vi "Test_Multiple_SubPanel_Self HSMO_External_Control.vi"() -> ()   [LabVIEW 2021]
uses:
  C:/Program Files (x86)/Hyper State Machine Framework/SSW_Hyper_State_Machine.lvlibp/State_Machine_Class/Main_State_Machine/Hyper_State_Machine.lvclass
  C:/Program Files (x86)/Hyper State Machine Framework/SSW_Hyper_State_Machine.lvlibp/State_Machine_Class/State_Machine_Module.llb/State Machine.ctl
  C:/Program Files (x86)/Hyper State Machine Framework/SSW_Hyper_State_Machine.lvlibp
panel:
  in  "Panel Index":i32
  in  "Change Mode":bool=TRUE
  out "Total_State":i32 caption="Total Independent State Object"
  in  "Show Stop Button":bool
  in  "UnLoad_Panel":bool
  in  "Load_Panel":bool
  in  "Time Target (s)":dbl=30.0 format="%#_13g"
  in  "System_Delay(s)":dbl=0.01 format="%.0p"
  in  "State_Interval_Time(s)":dbl format="%.0p"
  in  "State#":i32=100
  in  "Stop":bool=TRUE
  out "State[]":refnum<class "Hyper_State_Machine.lvclass">[][](array[class])
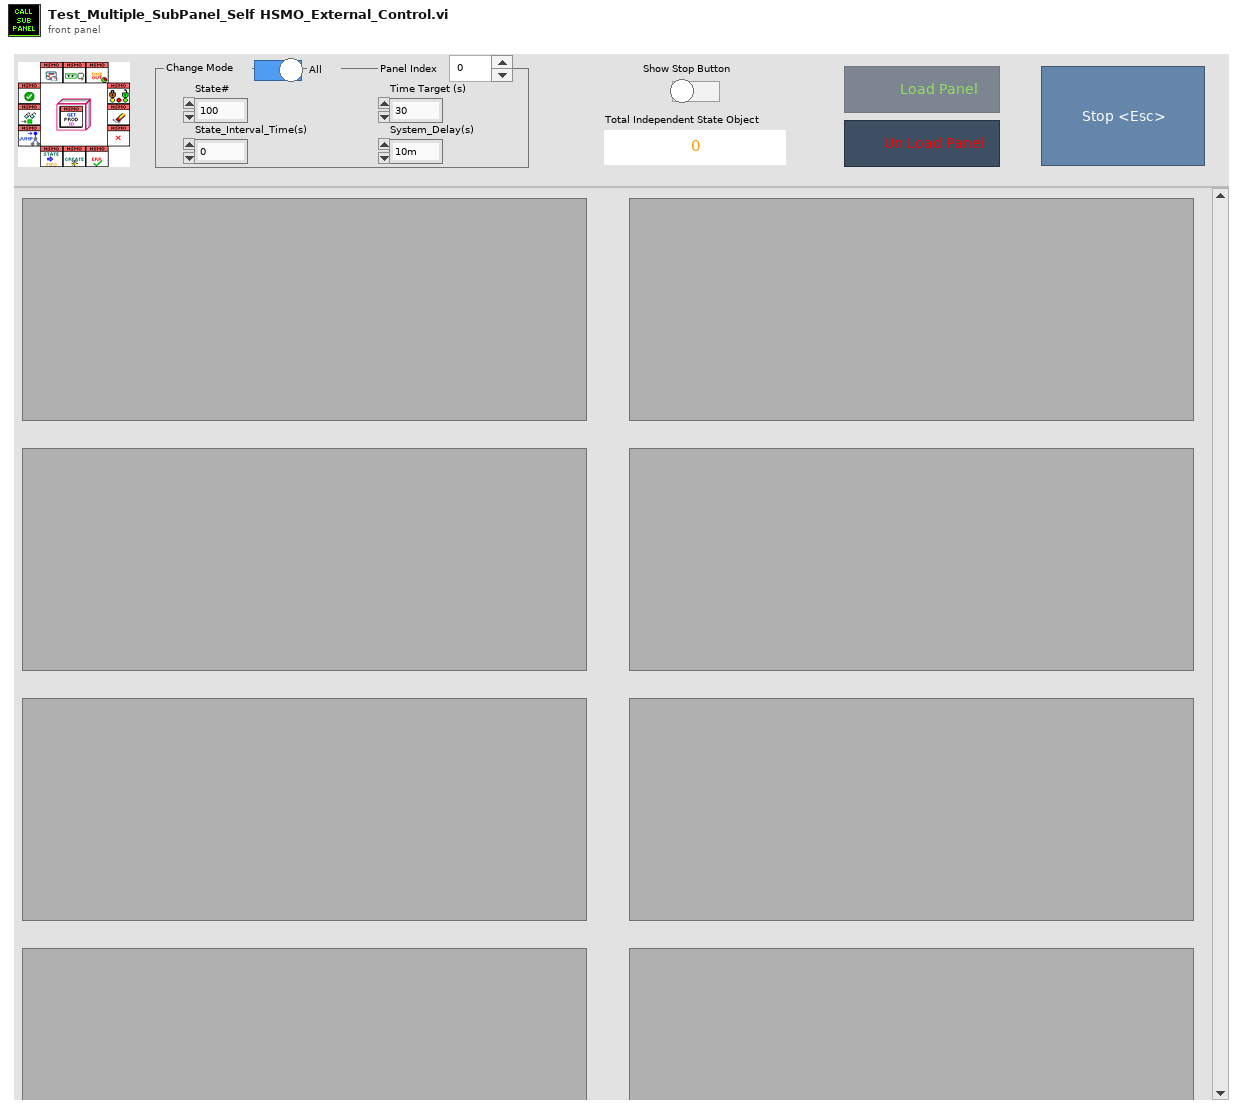
[diagram p1: front panel]
types:
  T1 = enum8{"Enabled", "Disabled", "Disabled and Grayed Out"}
  T2 = typedef "SSW_Hyper_State_Machine.lvlibp/State Machine.ctl" = cluster{"Command":string, "Data":variant}
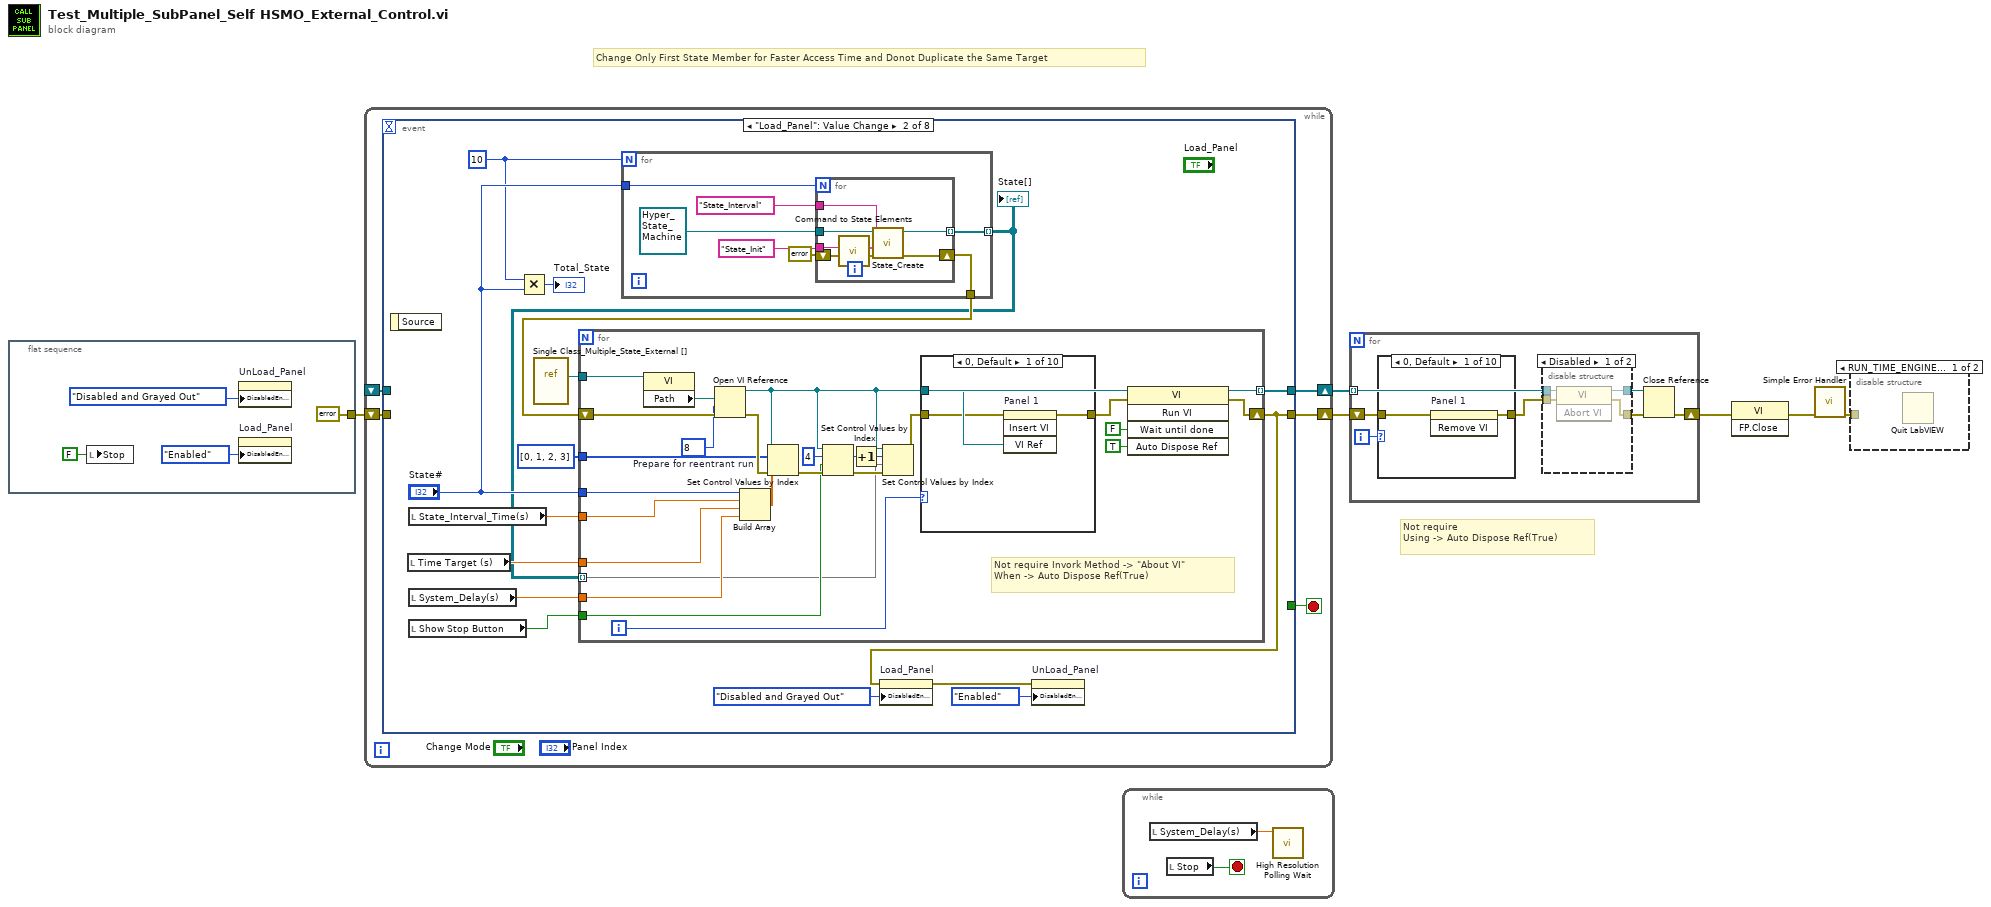
[diagram p0: block diagram]
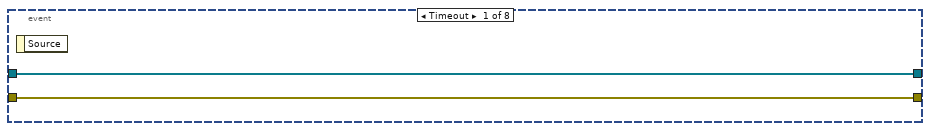
[diagram p3: hidden frame]
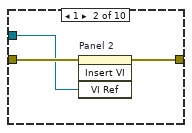
[diagram p4: hidden frame]
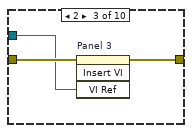
[diagram p5: hidden frame]
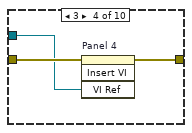
[diagram p6: hidden frame]
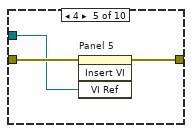
[diagram p7: hidden frame]
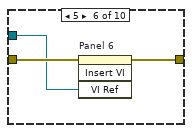
[diagram p8: hidden frame]
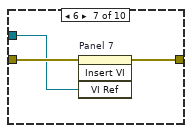
[diagram p9: hidden frame]
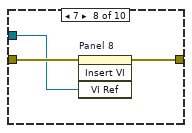
[diagram p10: hidden frame]
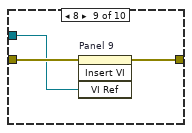
[diagram p11: hidden frame]
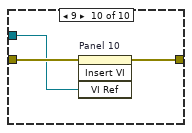
[diagram p12: hidden frame]
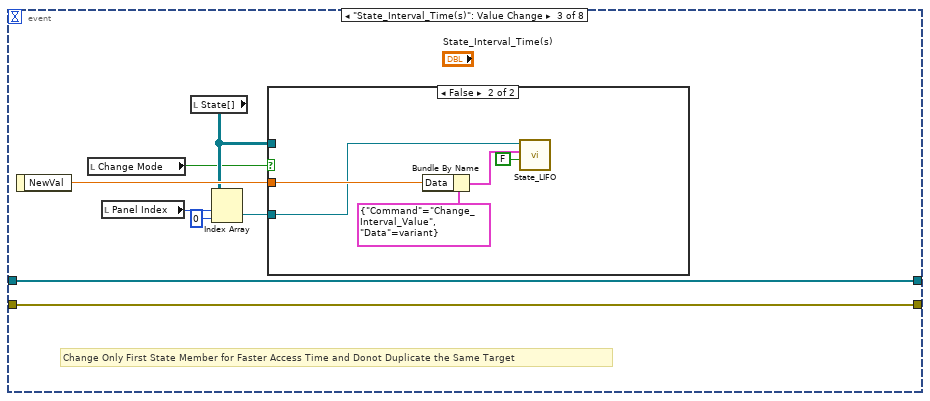
[diagram p13: hidden frame]
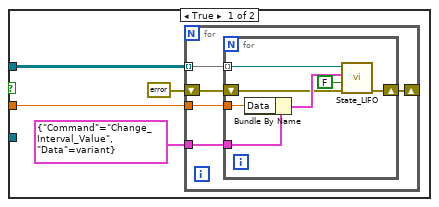
[diagram p14: hidden frame]
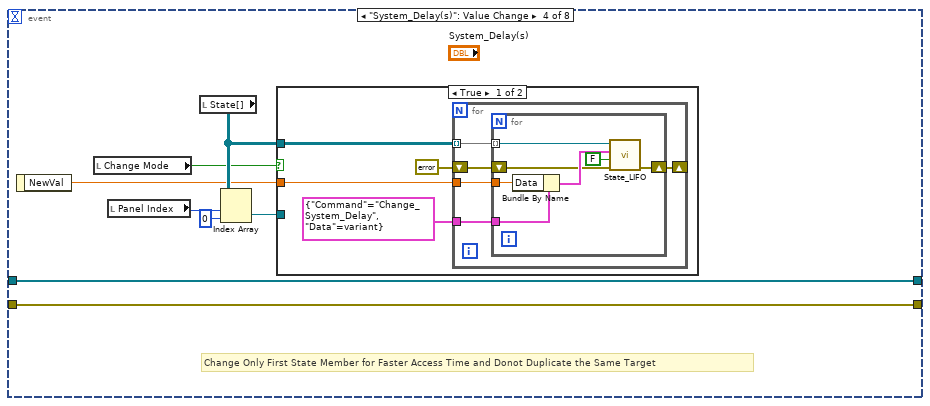
[diagram p15: hidden frame]
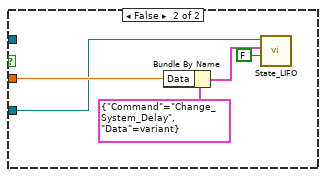
[diagram p16: hidden frame]
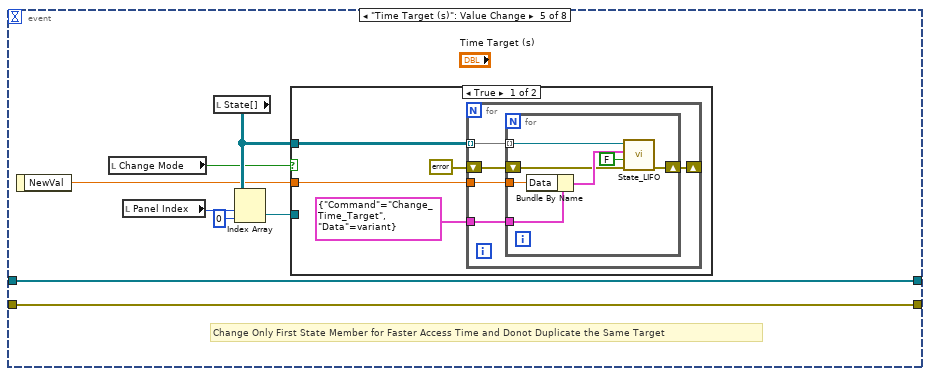
[diagram p17: hidden frame]
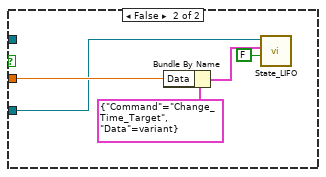
[diagram p18: hidden frame]
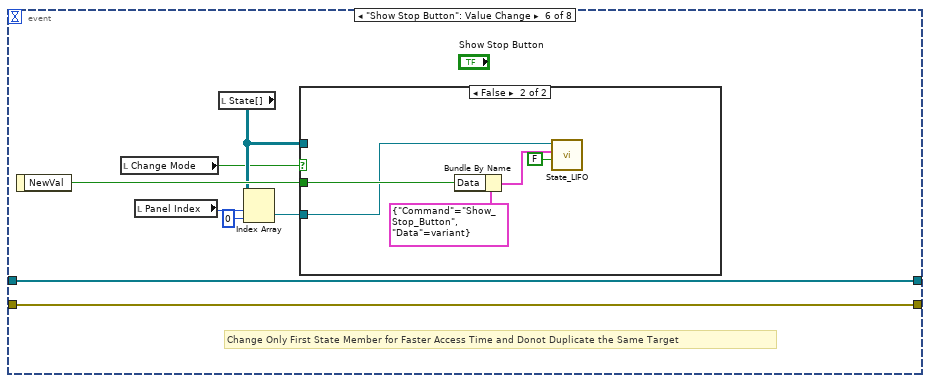
[diagram p19: hidden frame]
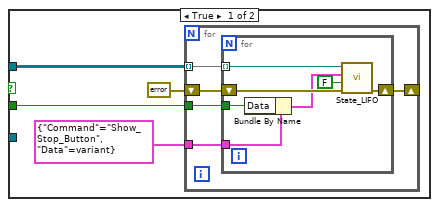
[diagram p20: hidden frame]
diagram:
  # "Change Only First State Member for Faster Access Time and Donot Duplicate the Same Target"
  # "Not require\nUsing -> Auto Dispose Ref(True)"
  n1 = flat-sequence {
    tunnel: [errorcluster {"status"=FALSE, "code"=0, "source"=""} ("error out")] -> w4
    frame #0 {
      n2 = local write "Stop"(FALSE ("Stop")) -> ()
      n3 = property on="UnLoad_Panel" class="Bool"("DisabledEnum"=T1."Disabled and Grayed Out" ("Disabled")) -> ()  [unwired: 2 in, 2 out]
      n4 = property on="Load_Panel" class="Bool"("DisabledEnum"=T1."Enabled" ("Disabled")) -> ()  [unwired: 2 in, 2 out]
    }
  }
  n5 = while {
    shift-right: [w14] -> w6
    shift-left: _ -> [w13]
    shift-right: [w12] -> w5
    shift-left: w4 -> [w11]
    stop <- w15 stop-if-true
    n6 = event shown="[1] \"Load_Panel\": Value Change" {
      selector: _ -> [_ _ _ _ _ _ _ _]
      dyn-events: _ -> [_ _ _ _ _ _ _ _]
      timeout: _ -> [_ _ _ _ _ _ _ _]
      tunnel: [_ _ _ _ _ _ _ w259] -> w15
      tunnel: [w17 w32 w109 w139 w168 w197 _ w260] -> w14
      tunnel: w13 -> [w17 _ w109 w139 w168 w197 w224 w260]
      tunnel: [w16 w28 w108 w138 w167 w196 _ w258] -> w12
      tunnel: w11 -> [w16 _ w108 w138 w167 w196 w220 w258]
      event Timeout {
        n7 = event-data() -> ()  [unwired: 1 in, 1 out]
      }
      event "Load_Panel": Value Change {
        w23 = 10
        n8 = event-data() -> ()  [unwired: 1 in, 1 out]
        n9 = local read "Time Target (s)"() -> (w20:dbl)
        n10 = local read "State_Interval_Time(s)"() -> (w26:dbl)
        n11 = local read "System_Delay(s)"() -> (w22:dbl)
        n12 = local read "Show Stop Button"() -> (w21:bool)
        n13 = Multiply(x=w23, y="State#") -> (x*y=→"Total_State":i32)
        n14 = vi-ref "Single Class_Multiple_State_External [].vi"() -> (w18:refnum<vi>)
        n15 = for {
          N: w23 -> [_]
          tunnel: [w36] -> w25
          tunnel: "State#" -> [w35]
          tunnel: [w34] -> w19 mode=indexing
          n16 = for {
            N: w35 -> [_]
            tunnel: refnum<class "Hyper_State_Machine.lvclass"> refnum ("SSW_Hyper_State_Machine.lvlibp:Hyper_State_Machine.lvclass") -> [w47]
            tunnel: "State_Init" ("Command") -> [w45]
            tunnel: "State_Interval" ("Core_Interval_Name(State_Interval)") -> [w44]
            shift-right: [w43] -> w36
            shift-left: errorcluster {"status"=FALSE, "code"=0, "source"=""} ("error out") -> [w42]
            tunnel: [w41] -> w34 mode=indexing
            n17 = call "Command to State Elements.vi"("Command"=w45) -> ("Command to State Elements"=w46:T2)  [unwired: 10 in]
            n18 = call-dynamic "State_Create.vi"("error in (no error)"=w42, "Init_State(Option)"=w46, "State_Interval_Name"=w44, "State_Machine_Class in"=w47) -> ("error out"=w43:errorcluster, "State_Machine_Class out"=w41:refnum<class "Hyper_State_Machine.lvclass">)  [unwired: 5 in, 1 out]
          }
        }
        "State[]" <- w19
        n19 = for {
          shift-right: [w65] -> w28
          shift-left: w25 -> [w71]
          tunnel: [w67] -> w32 mode=indexing
          tunnel: w26 -> [w62]
          tunnel: "State#" -> [w61]
          tunnel: w22 -> [w60]
          tunnel: w20 -> [w59]
          tunnel: i32[] [0, 1, 2, 3] ("control indexes") -> [w58]
          tunnel: w21 -> [w57]
          tunnel: w19 -> [w50] mode=indexing
          tunnel: w18 -> [w48]
          i -> [w51]
          w54 = 4
          w49 = 8  # Prepare for reentrant run
          # "Not require Invork Method -> \"About VI\"\nWhen -> Auto Dispose Ref(True)"
          n20 = property class="VI"(reference=w48) -> ("Path"=w72:path)  [unwired: 1 in, 2 out]
          n21 = Open VI Reference(vi path=w72, options=w49, error in (no error)=w71) -> (vi reference=w52:refnum<vi>, error out=w70:errorcluster)  [unwired: 3 in]
          n22 = Build Array(w61, w62, w59, w60) -> (w64:dbl[])
          n23 = Set Control Values by Index(0:w52, 1:w58, 2:w64, 3:w70) -> (11:w63:errorcluster)
          n24 = Set Control Values by Index(0:w52, 1:w54, 2:w57, 3:w63) -> (11:w56:errorcluster)
          n25 = Increment(x=w54) -> (x+1=w53:i32)
          n26 = Set Control Values by Index(0:w52, 1:w53, 2:w50, 3:w56) -> (11:w55:errorcluster)
          n27 = case shown="0, Default" w51 {
            tunnel: w55 -> [w73 w78 w81 w84 w87 w90 w93 w96 w99 w102]
            tunnel: w52 -> [w74 w77 w79 w82 w85 w88 w91 w94 w97 w100]
            tunnel: [w75 w76 w80 w83 w86 w89 w92 w95 w98 w101] -> w66
            frame 0, Default {
              n28 = invoke on="Panel 1" class="SubPnl" method="Insert VI"(error in=w73, "VI Ref"=w74) -> (error out=w75:errorcluster)  [unwired: 2 in, 3 out]
            }
            frame 1 {
              n29 = invoke on="Panel 2" class="SubPnl" method="Insert VI"(error in=w78, "VI Ref"=w77) -> (error out=w76:errorcluster)  [unwired: 2 in, 3 out]
            }
            frame 2 {
              n30 = invoke on="Panel 3" class="SubPnl" method="Insert VI"(error in=w81, "VI Ref"=w79) -> (error out=w80:errorcluster)  [unwired: 2 in, 3 out]
            }
            frame 3 {
              n31 = invoke on="Panel 4" class="SubPnl" method="Insert VI"(error in=w84, "VI Ref"=w82) -> (error out=w83:errorcluster)  [unwired: 2 in, 3 out]
            }
            frame 4 {
              n32 = invoke on="Panel 5" class="SubPnl" method="Insert VI"(error in=w87, "VI Ref"=w85) -> (error out=w86:errorcluster)  [unwired: 2 in, 3 out]
            }
            frame 5 {
              n33 = invoke on="Panel 6" class="SubPnl" method="Insert VI"(error in=w90, "VI Ref"=w88) -> (error out=w89:errorcluster)  [unwired: 2 in, 3 out]
            }
            frame 6 {
              n34 = invoke on="Panel 7" class="SubPnl" method="Insert VI"(error in=w93, "VI Ref"=w91) -> (error out=w92:errorcluster)  [unwired: 2 in, 3 out]
            }
            frame 7 {
              n35 = invoke on="Panel 8" class="SubPnl" method="Insert VI"(error in=w96, "VI Ref"=w94) -> (error out=w95:errorcluster)  [unwired: 2 in, 3 out]
            }
            frame 8 {
              n36 = invoke on="Panel 9" class="SubPnl" method="Insert VI"(error in=w99, "VI Ref"=w97) -> (error out=w98:errorcluster)  [unwired: 2 in, 3 out]
            }
            frame 9 {
              n37 = invoke on="Panel 10" class="SubPnl" method="Insert VI"(error in=w102, "VI Ref"=w100) -> (error out=w101:errorcluster)  [unwired: 2 in, 3 out]
            }
          }
          n38 = invoke class="VI" method="Run VI"(reference=w52, error in=w66, "Wait until done"=FALSE ("Wait Until Done"), "Auto Dispose Ref"=TRUE ("Auto Dispose Reference")) -> (reference out=w67:refnum<vi>, error out=w65:errorcluster)  [unwired: 1 in, 3 out]
        }
        n39 = property on="Load_Panel" class="Bool"(error in=w28, "DisabledEnum"=T1."Disabled and Grayed Out" ("Disabled")) -> (error out=w29:errorcluster)  [unwired: 1 in, 1 out]
        n40 = property on="UnLoad_Panel" class="Bool"(error in=w29, "DisabledEnum"=T1."Enabled" ("Disabled")) -> ()  [unwired: 1 in, 2 out]
      }
      event "State_Interval_Time(s)": Value Change {
        # "Change Only First State Member for Faster Access Time and Donot Duplicate the Same Target"
        n41 = event-data() -> ("NewVal"=w110:dbl)  [unwired: 1 in]
        n42 = local read "Change Mode"() -> (w104:bool)
        n43 = local read "Panel Index"() -> (w103:i32)
        n44 = local read "State[]"() -> (w107:refnum<class "Hyper_State_Machine.lvclass">[][])
        n45 = Index Array(array=w107, index (row)=w103, index (col)=0 ("disabled index (col)")) -> (element=w106:refnum<class "Hyper_State_Machine.lvclass">)
        n46 = case shown="False" w104 {
          tunnel: w110 -> [w114 w131]
          tunnel: w107 -> [w111 _]
          tunnel: w106 -> [_ w130]
          frame True {
            n47 = for {
              tunnel: w111 -> [w119] mode=indexing
              shift-right: [w116] -> _
              shift-left: errorcluster {"status"=FALSE, "code"=0, "source"=""} ("error out") -> [w117]
              tunnel: w114 -> [w118]
              tunnel: T2 {"Command"="Change_Interval_Value", "Data"=variant} ("State Machine") -> [w115]
              n48 = for {
                tunnel: w119 -> [w122] mode=indexing
                tunnel: w118 -> [w125]
                shift-right: [w124] -> w116
                shift-left: w117 -> [w121]
                tunnel: w115 -> [w123]
                n49 = Bundle By Name(cluster=w123, "Data"=w125) -> (w126:T2)
                n50 = call-dynamic "State_LIFO.vi"("error in (no error)"=w121, "State_Interval(Enable)"=FALSE, "State Machine"=w126, "State_Machine_Class in"=w122) -> ("error out"=w124:errorcluster)  [unwired: 6 in, 1 out]
              }
            }
          }
          frame False {
            n51 = Bundle By Name(cluster=T2 {"Command"="Change_Interval_Value", "Data"=variant} ("State Machine"), "Data"=w131) -> (w128:T2)
            n52 = call-dynamic "State_LIFO.vi"("State_Interval(Enable)"=FALSE, "State Machine"=w128, "State_Machine_Class in"=w130) -> ()  [unwired: 7 in, 2 out]
          }
        }
      }
      event "System_Delay(s)": Value Change {
        # "Change Only First State Member for Faster Access Time and Donot Duplicate the Same Target"
        n53 = event-data() -> ("NewVal"=w135:dbl)  [unwired: 1 in]
        n54 = local read "Change Mode"() -> (w133:bool)
        n55 = local read "Panel Index"() -> (w132:i32)
        n56 = local read "State[]"() -> (w137:refnum<class "Hyper_State_Machine.lvclass">[][])
        n57 = Index Array(array=w137, index (row)=w132, index (col)=0 ("disabled index (col)")) -> (element=w136:refnum<class "Hyper_State_Machine.lvclass">)
        n58 = case shown="True" w133 {
          tunnel: w135 -> [w143 w160]
          tunnel: w137 -> [w140 _]
          tunnel: w136 -> [_ w159]
          frame True {
            n59 = for {
              tunnel: w140 -> [w148] mode=indexing
              shift-right: [w145] -> _
              shift-left: errorcluster {"status"=FALSE, "code"=0, "source"=""} ("error out") -> [w146]
              tunnel: w143 -> [w147]
              tunnel: T2 {"Command"="Change_System_Delay", "Data"=variant} ("State Machine") -> [w144]
              n60 = for {
                tunnel: w148 -> [w151] mode=indexing
                tunnel: w147 -> [w154]
                shift-right: [w153] -> w145
                shift-left: w146 -> [w150]
                tunnel: w144 -> [w152]
                n61 = Bundle By Name(cluster=w152, "Data"=w154) -> (w155:T2)
                n62 = call-dynamic "State_LIFO.vi"("error in (no error)"=w150, "State_Interval(Enable)"=FALSE, "State Machine"=w155, "State_Machine_Class in"=w151) -> ("error out"=w153:errorcluster)  [unwired: 6 in, 1 out]
              }
            }
          }
          frame False {
            n63 = Bundle By Name(cluster=T2 {"Command"="Change_System_Delay", "Data"=variant} ("State Machine"), "Data"=w160) -> (w157:T2)
            n64 = call-dynamic "State_LIFO.vi"("State_Interval(Enable)"=FALSE, "State Machine"=w157, "State_Machine_Class in"=w159) -> ()  [unwired: 7 in, 2 out]
          }
        }
      }
      event "Time Target (s)": Value Change {
        # "Change Only First State Member for Faster Access Time and Donot Duplicate the Same Target"
        n65 = event-data() -> ("NewVal"=w164:dbl)  [unwired: 1 in]
        n66 = local read "Change Mode"() -> (w162:bool)
        n67 = local read "Panel Index"() -> (w161:i32)
        n68 = local read "State[]"() -> (w166:refnum<class "Hyper_State_Machine.lvclass">[][])
        n69 = Index Array(array=w166, index (row)=w161, index (col)=0 ("disabled index (col)")) -> (element=w165:refnum<class "Hyper_State_Machine.lvclass">)
        n70 = case shown="True" w162 {
          tunnel: w164 -> [w172 w189]
          tunnel: w166 -> [w169 _]
          tunnel: w165 -> [_ w188]
          frame True {
            n71 = for {
              tunnel: w169 -> [w177] mode=indexing
              shift-right: [w174] -> _
              shift-left: errorcluster {"status"=FALSE, "code"=0, "source"=""} ("error out") -> [w175]
              tunnel: w172 -> [w176]
              tunnel: T2 {"Command"="Change_Time_Target", "Data"=variant} ("State Machine") -> [w173]
              n72 = for {
                tunnel: w177 -> [w180] mode=indexing
                tunnel: w176 -> [w183]
                shift-right: [w182] -> w174
                shift-left: w175 -> [w179]
                tunnel: w173 -> [w181]
                n73 = Bundle By Name(cluster=w181, "Data"=w183) -> (w184:T2)
                n74 = call-dynamic "State_LIFO.vi"("error in (no error)"=w179, "State_Interval(Enable)"=FALSE, "State Machine"=w184, "State_Machine_Class in"=w180) -> ("error out"=w182:errorcluster)  [unwired: 6 in, 1 out]
              }
            }
          }
          frame False {
            n75 = Bundle By Name(cluster=T2 {"Command"="Change_Time_Target", "Data"=variant} ("State Machine"), "Data"=w189) -> (w186:T2)
            n76 = call-dynamic "State_LIFO.vi"("State_Interval(Enable)"=FALSE, "State Machine"=w186, "State_Machine_Class in"=w188) -> ()  [unwired: 7 in, 2 out]
          }
        }
      }
      event "Show Stop Button": Value Change {
        # "Change Only First State Member for Faster Access Time and Donot Duplicate the Same Target"
        n77 = event-data() -> ("NewVal"=w194:bool)  [unwired: 1 in]
        n78 = local read "Change Mode"() -> (w191:bool)
        n79 = local read "Panel Index"() -> (w190:i32)
        n80 = local read "State[]"() -> (w192:refnum<class "Hyper_State_Machine.lvclass">[][])
        n81 = Index Array(array=w192, index (row)=w190, index (col)=0 ("disabled index (col)")) -> (element=w195:refnum<class "Hyper_State_Machine.lvclass">)
        n82 = case shown="False" w191 {
          tunnel: w194 -> [w201 w218]
          tunnel: w195 -> [_ w217]
          tunnel: w192 -> [w198 _]
          frame True {
            n83 = for {
              tunnel: w198 -> [w206] mode=indexing
              shift-right: [w203] -> _
              shift-left: errorcluster {"status"=FALSE, "code"=0, "source"=""} ("error out") -> [w204]
              tunnel: w201 -> [w205]
              tunnel: T2 {"Command"="Show_Stop_Button", "Data"=variant} ("State Machine") -> [w202]
              n84 = for {
                tunnel: w206 -> [w213] mode=indexing
                tunnel: w205 -> [w212]
                tunnel: w202 -> [w209]
                shift-right: [w210] -> w203
                shift-left: w204 -> [w211]
                n85 = Bundle By Name(cluster=w209, "Data"=w212) -> (w208:T2)
                n86 = call-dynamic "State_LIFO.vi"("error in (no error)"=w211, "State_Interval(Enable)"=FALSE, "State Machine"=w208, "State_Machine_Class in"=w213) -> ("error out"=w210:errorcluster)  [unwired: 6 in, 1 out]
              }
            }
          }
          frame False {
            n87 = Bundle By Name(cluster=T2 {"Command"="Show_Stop_Button", "Data"=variant} ("State Machine"), "Data"=w218) -> (w215:T2)
            n88 = call-dynamic "State_LIFO.vi"("State_Interval(Enable)"=FALSE, "State Machine"=w215, "State_Machine_Class in"=w217) -> ()  [unwired: 7 in, 2 out]
          }
        }
      }
      event "UnLoad_Panel": Value Change {
        # "Do not using Shift Register to ignore some case Error"
        # "Not require\nUsing -> Auto Dispose Ref(True)"
        n89 = event-data() -> ()  [unwired: 1 in, 1 out]
        n90 = for {
          tunnel: w224 -> [w229] mode=indexing
          tunnel: w220 -> [w226]
          tunnel: [w225] -> w219
          i -> [w228]
          n91 = case shown="0, Default" w228 {
            tunnel: w226 -> [w238 w241 w243 w245 w247 w249 w251 w253 w255 w257]
            tunnel: w229 -> [_ _ _ _ _ _ _ _ _ _]
            tunnel: [w239 w240 w242 w244 w246 w248 w250 w252 w254 w256] -> w227
            frame 0, Default {
              n92 = invoke on="Panel 1" class="SubPnl" method="Remove VI"(error in=w238) -> (error out=w239:errorcluster)  [unwired: 2 in, 2 out]
            }
            frame 1 {
              n93 = invoke on="Panel 2" class="SubPnl" method="Remove VI"(error in=w241) -> (error out=w240:errorcluster)  [unwired: 2 in, 2 out]
            }
            frame 2 {
              n94 = invoke on="Panel 3" class="SubPnl" method="Remove VI"(error in=w243) -> (error out=w242:errorcluster)  [unwired: 2 in, 2 out]
            }
            frame 3 {
              n95 = invoke on="Panel 4" class="SubPnl" method="Remove VI"(error in=w245) -> (error out=w244:errorcluster)  [unwired: 2 in, 2 out]
            }
            frame 4 {
              n96 = invoke on="Panel 5" class="SubPnl" method="Remove VI"(error in=w247) -> (error out=w246:errorcluster)  [unwired: 2 in, 2 out]
            }
            frame 5 {
              n97 = invoke on="Panel 6" class="SubPnl" method="Remove VI"(error in=w249) -> (error out=w248:errorcluster)  [unwired: 2 in, 2 out]
            }
            frame 6 {
              n98 = invoke on="Panel 7" class="SubPnl" method="Remove VI"(error in=w251) -> (error out=w250:errorcluster)  [unwired: 2 in, 2 out]
            }
            frame 7 {
              n99 = invoke on="Panel 8" class="SubPnl" method="Remove VI"(error in=w253) -> (error out=w252:errorcluster)  [unwired: 2 in, 2 out]
            }
            frame 8 {
              n100 = invoke on="Panel 9" class="SubPnl" method="Remove VI"(error in=w255) -> (error out=w254:errorcluster)  [unwired: 2 in, 2 out]
            }
            frame 9 {
              n101 = invoke on="Panel 10" class="SubPnl" method="Remove VI"(error in=w257) -> (error out=w256:errorcluster)  [unwired: 2 in, 2 out]
            }
          }
          n102 = disable-structure shown="Enabled" {
            disable-tunnel: [w235 w237] -> w231
            disable-tunnel: [w234 w236] -> w230
            disable-tunnel: w229 -> [w233 w237]
            disable-tunnel: w227 -> [w232 w236]
            frame Disabled {
              n103 = invoke class="VI" method="Abort VI"(reference=w233, error in=w232) -> (reference out=w235:refnum<vi>, error out=w234:errorcluster)  [unwired: 1 in, 1 out]
            }
            frame Enabled {
            }
          }
          n104 = Close Reference(reference=w231, error in (no error)=w230) -> (error out=w225:errorcluster)
        }
        n105 = property on="UnLoad_Panel" class="Bool"(error in=w219, "DisabledEnum"=T1."Disabled and Grayed Out" ("Disabled")) -> (error out=w221:errorcluster)  [unwired: 1 in, 1 out]
        n106 = property on="Load_Panel" class="Bool"(error in=w221, "DisabledEnum"=T1."Enabled" ("Disabled")) -> ()  [unwired: 1 in, 2 out]
      }
      event "Stop": Value Change {
        n107 = event-data() -> ()  [unwired: 1 in, 1 out]
        n108 = Two Button Dialog(message="Exit Confirm !") -> (T button?=w259:bool)  [unwired: 2 in]
        n109 = local write "Stop"(w259) -> ()
      }
    }
  }
  n110 = while {
    stop <- w262 stop-if-true
    n111 = local read "System_Delay(s)"() -> (w263:dbl)
    n112 = local read "Stop"() -> (w262:bool)
    n113 = call <vilib>:"High Resolution Polling Wait.vi"("seconds to wait"=w263) -> ()  [unwired: 10 in, 1 out]
  }
  n114 = for {
    tunnel: w6 -> [w270] mode=indexing
    shift-right: [w267] -> w2
    shift-left: w5 -> [w266]
    i -> [w265]
    n115 = case shown="0, Default" w265 {
      tunnel: w266 -> [w277 w280 w282 w284 w286 w288 w290 w292 w294 w296]
      tunnel: [w278 w279 w281 w283 w285 w287 w289 w291 w293 w295] -> w264
      frame 0, Default {
        n116 = invoke on="Panel 1" class="SubPnl" method="Remove VI"(error in=w277) -> (error out=w278:errorcluster)  [unwired: 2 in, 2 out]
      }
      frame 1 {
        n117 = invoke on="Panel 2" class="SubPnl" method="Remove VI"(error in=w280) -> (error out=w279:errorcluster)  [unwired: 2 in, 2 out]
      }
      frame 2 {
        n118 = invoke on="Panel 3" class="SubPnl" method="Remove VI"(error in=w282) -> (error out=w281:errorcluster)  [unwired: 2 in, 2 out]
      }
      frame 3 {
        n119 = invoke on="Panel 4" class="SubPnl" method="Remove VI"(error in=w284) -> (error out=w283:errorcluster)  [unwired: 2 in, 2 out]
      }
      frame 4 {
        n120 = invoke on="Panel 5" class="SubPnl" method="Remove VI"(error in=w286) -> (error out=w285:errorcluster)  [unwired: 2 in, 2 out]
      }
      frame 5 {
        n121 = invoke on="Panel 6" class="SubPnl" method="Remove VI"(error in=w288) -> (error out=w287:errorcluster)  [unwired: 2 in, 2 out]
      }
      frame 6 {
        n122 = invoke on="Panel 7" class="SubPnl" method="Remove VI"(error in=w290) -> (error out=w289:errorcluster)  [unwired: 2 in, 2 out]
      }
      frame 7 {
        n123 = invoke on="Panel 8" class="SubPnl" method="Remove VI"(error in=w292) -> (error out=w291:errorcluster)  [unwired: 2 in, 2 out]
      }
      frame 8 {
        n124 = invoke on="Panel 9" class="SubPnl" method="Remove VI"(error in=w294) -> (error out=w293:errorcluster)  [unwired: 2 in, 2 out]
      }
      frame 9 {
        n125 = invoke on="Panel 10" class="SubPnl" method="Remove VI"(error in=w296) -> (error out=w295:errorcluster)  [unwired: 2 in, 2 out]
      }
    }
    n126 = disable-structure shown="Disabled" {
      disable-tunnel: w270 -> [w274 w276]
      disable-tunnel: [w273 w276] -> w269
      disable-tunnel: [w272 w275] -> w268
      disable-tunnel: w264 -> [w271 w275]
      frame Disabled {
        n127 = invoke class="VI" method="Abort VI"(reference=w274, error in=w271) -> (reference out=w273:refnum<vi>, error out=w272:errorcluster)  [unwired: 1 in, 1 out]
      }
      frame Enabled {
      }
    }
    n128 = Close Reference(reference=w269, error in (no error)=w268) -> (error out=w267:errorcluster)
  }
  n129 = invoke class="VI" method="FP.Close"(error in=w2) -> (error out=w3:errorcluster)  [unwired: 2 in, 2 out]
  n130 = call <vilib>:"Simple Error Handler.vi"("error in (no error)"=w3) -> ("error out"=w1:errorcluster)  [unwired: 4 in, 4 out]
  n131 = disable-structure shown="RUN_TIME_ENGINE==True" {
    disable-tunnel: w1 -> [_ _]
    frame condition #0 {
      n132 = Quit LabVIEW() -> ()  [unwired: 1 in]
    }
    frame condition #1 (active) {
    }
  }
